vi "Set Window Title.vi"(0 "VI in":refnum<vi>, 11 "error in (no error)":errorcluster) -> (15 "error out":errorcluster)   [LabVIEW 2015]
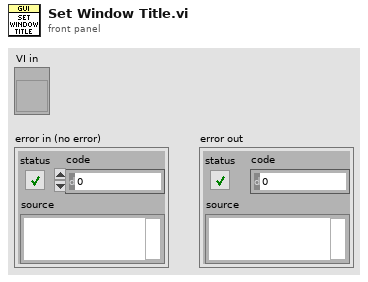
[diagram p1: front panel]
types:
  T1 = enum32{"invalid app kind", "Development System", "Run Time System", "Student Edition", "Embedded LabVIEW", "Evaluation", "Custom"}
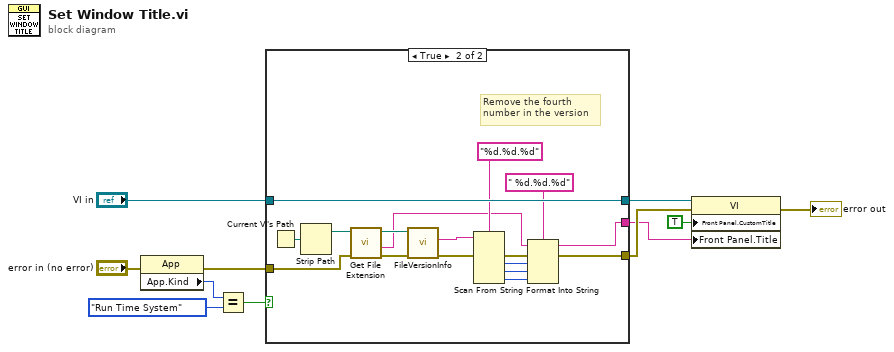
[diagram p0: block diagram]
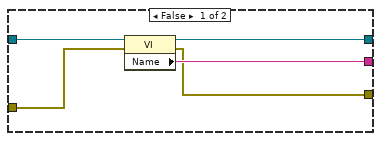
[diagram p2: hidden frame]
diagram:
  n1 = property class="App"(error in="error in (no error)") -> (error out=w5:errorcluster, "App.Kind"=w1:T1)  [unwired: 1 in, 1 out]
  n2 = Equal?(x=w1, y=T1."Run Time System" ("Application:Kind")) -> (x = y?=w3:bool)
  n3 = case shown="True" w3 {
    tunnel: [w16 w17] -> w8
    tunnel: w5 -> [w15 w29]
    tunnel: [w14 w21] -> w9
    tunnel: "VI in" -> [w13 w28]
    tunnel: [w12 w28] -> w7
    frame False {
      n4 = property class="VI"(reference=w13, error in=w15) -> (reference out=w12:refnum<vi>, error out=w14:errorcluster, "Name"=w16:string)
    }
    frame True {
      # "Remove the fourth\nnumber in the version"
      n5 = Current VI's Path() -> (path=w33:path)
      n6 = Strip Path(path=w33) -> (stripped path=w32:path)  [unwired: 1 out]
      n7 = call <vilib>:"Get File Extension.vi"("error in (no error)"=w29, "file"=w32) -> ("error out"=w30:errorcluster, "filename without extension"=w18:string, "dup file"=w31:path)  [unwired: 5 in, 2 out]
      n8 = call <vilib>:"FileVersionInfo.vi"("error in (no error)"=w30, "Application Path in"=w31) -> ("error out"=w22:errorcluster, "File Version Info"=w20:string)  [unwired: 6 in, 2 out]
      n9 = Scan From String(format string="%d.%d.%d", input string=w20, error in=w22) -> (error out=w23:errorcluster, output 1=w26:i32, output 2=w25:i32, output 3=w24:i32)  [unwired: 4 in, 2 out]
      n10 = Format Into String(format string=" %d.%d.%d", initial string=w18, error in=w23, w26, w25, w24) -> (resulting string=w17:string, error out=w21:errorcluster)
    }
  }
  n11 = property class="VI"(reference=w7, error in=w9, "Front Panel.CustomTitle"=TRUE ("Front Panel Window:Custom Title"), "Front Panel.Title"=w8) -> (error out=→"error out":errorcluster)  [unwired: 1 out]
